vi "Update Index Highlight.vi"(7 "Max Index":i32, 8 "Error In":errorcluster, 9 "UI control refnums":T1, 10 "Old Index":i32, 11 "New Index":i32) -> (0 "Error Out":errorcluster)   [LabVIEW 2012]
uses:
  Custom Controls and Typedefs/Macro_MD_UI Control Refnums.ctl
  Custom Controls and Typedefs/Delete Button.ctl
  Custom Controls and Typedefs/Edit Button.ctl
  SubVIs/FormatTree&TableStyle_Commands.ctl
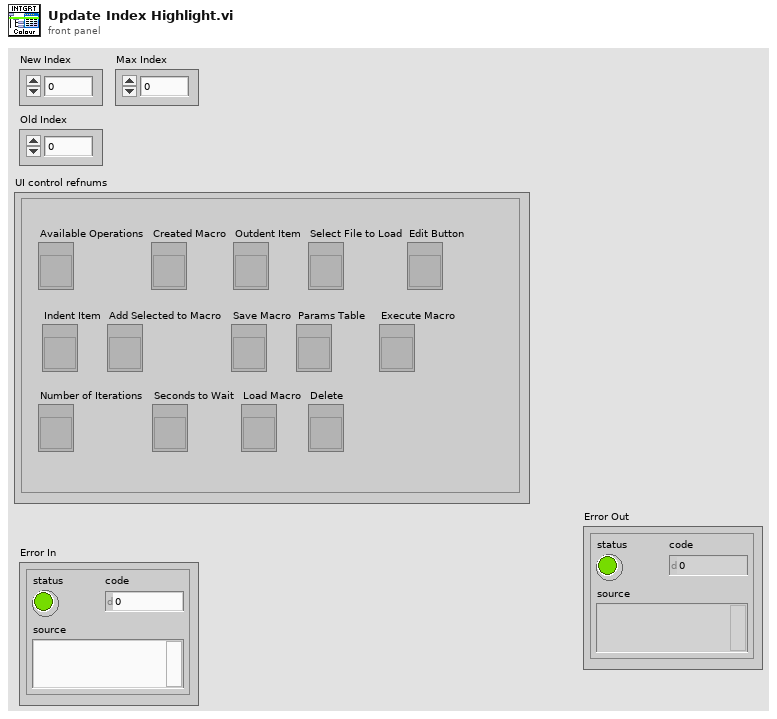
[diagram p1: front panel]
types:
  T1 = typedef "Macro_MD_UI Control Refnums.ctl" = cluster{"Available Operations":refnum<vi>, "Created Macro":refnum<vi>, "Indent Item":refnum<vi>, "Add Selected to Macro":refnum<vi>, "Outdent Item":refnum<vi>, "Number of Iterations":refnum<vi>, "Seconds to Wait":refnum<vi>, "Load Macro":refnum<vi>, "Save Macro":refnum<vi>, "Select File to Load":refnum<vi>, "Params Table":refnum<vi>, "Delete":refnum<vi>, "Edit Button":refnum<vi>, "Execute Macro":refnum<vi>}
  T2 = typedef "FormatTree&TableStyle_Commands.ctl" = enum16{"Colour Row", "Uncolour Row", "Bold Row", "Unbold Row", "Clear", "UpdateVisibleRows"}
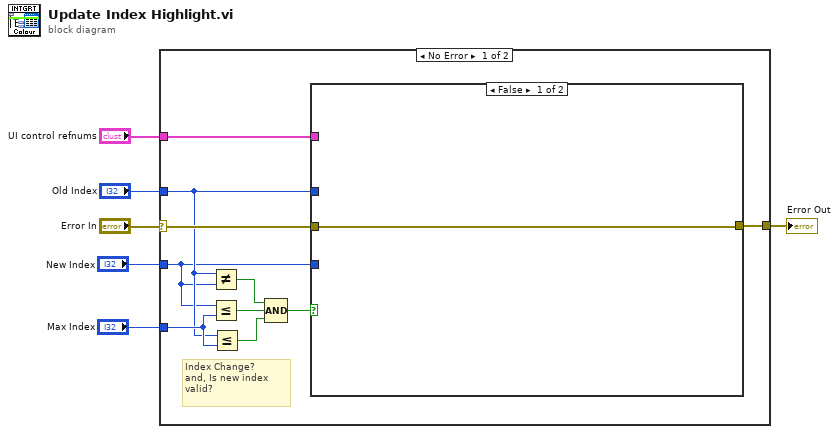
[diagram p0: block diagram]
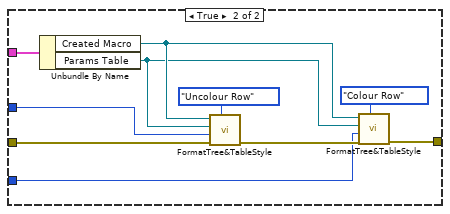
[diagram p2: hidden frame]
diagram:
  n1 = case shown="No Error" "Error In" {
    selector: "Error In" -> [w15 w28]
    tunnel: "UI control refnums" -> [w16 _]
    tunnel: "Old Index" -> [w12 _]
    tunnel: "New Index" -> [w11 _]
    tunnel: [w14 w28] -> w2
    tunnel: "Max Index" -> [w13 _]
    frame No Error {
      # "Index Change?\nand, Is new index valid?"
      n2 = Not Equal?(x=w12, y=w11) -> (x != y?=w10:bool)
      n3 = Less Or Equal?(x=w11, y=w13) -> (x <= y?=w9:bool)
      n4 = Less Or Equal?(x=w12, y=w13) -> (x <= y?=w8:bool)
      n5 = Compound Arithmetic op=AND(w10, w9, w8) -> (w7:bool)
      n6 = case shown="False" w7 {
        tunnel: w16 -> [_ w27]
        tunnel: w12 -> [_ w21]
        tunnel: w15 -> [w17 w20]
        tunnel: w11 -> [_ w19]
        tunnel: [w17 w18] -> w14
        frame False {
        }
        frame True {
          n7 = Unbundle By Name(w27) -> ("Created Macro"=w24:refnum<vi>, "Params Table"=w23:refnum<vi>)
          n8 = call "FormatTree&TableStyle.vi"("Format Command"=FormatTree&TableStyle_Commands."Uncolour Row", "Error In"=w20, "Row Index"=w21, "Tbl Refnum"=w23, "Tree Refnum"=w24) -> ("Error Out"=w22:errorcluster)  [unwired: 6 in]
          n9 = call "FormatTree&TableStyle.vi"("Format Command"=FormatTree&TableStyle_Commands."Colour Row", "Error In"=w22, "Row Index"=w19, "Tbl Refnum"=w23, "Tree Refnum"=w24) -> ("Error Out"=w18:errorcluster)  [unwired: 6 in]
        }
      }
    }
    frame Error {
    }
  }
  "Error Out" <- w2
